vi "niSYS - SA - MEAS - UTIL - 1 Ohm Voltage to dBm (CSGL array).vi"(7 "Complex Array, V":cdb[](array[numeric]) format="%.1f") -> (8 "Real Array, dBm":dbl[](array[numeric]) format="%.3f")   [LabVIEW 2019]
doc: "(c) Copyright 2006, National Instruments, Inc. This VI may not be duplicated, sold, or distributed without written consent from National Instruments."
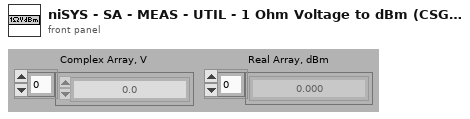
[diagram p1: front panel]
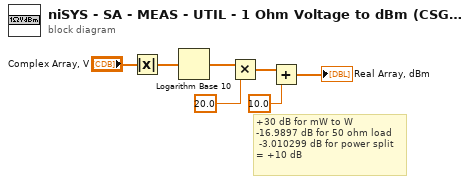
[diagram p0: block diagram]
diagram:
  # "+30 dB for mW to W\n-16.9897 dB for 50 ohm load\n -3.010299 dB for power split\n= +10 dB"
  n1 = Absolute Value(x="Complex Array, V") -> (abs(x)=w4:dbl[])
  n2 = Logarithm Base 10(1:w4) -> (0:w6:dbl[])
  n3 = Multiply(x=w6, y=20.0) -> (x*y=w5:dbl[])
  n4 = Add(x=w5, y=10.0) -> (x+y=→"Real Array, dBm":dbl[])
